vi "manual_trigger.vi"() -> ()   [LabVIEW 2011]
panel:
  in  "double trigger fast":bool
  in  "meas delay":u32
  in  "double trigger delayed":bool
  out "trigger number":i32
  in  "cont. trigger":bool
  in  "milliseconds to wait":u32=100
  in  "number of triggers":i32
  in  "single trigger":bool
  in  "stop":bool
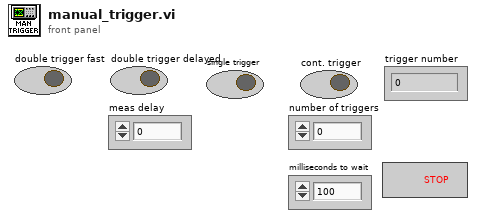
[diagram p1: front panel]
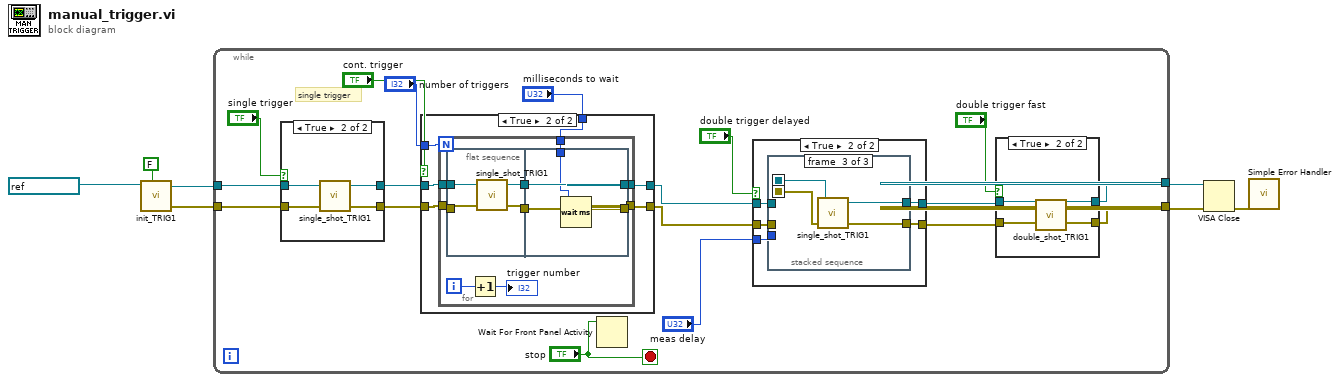
[diagram p0: block diagram]
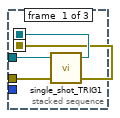
[diagram p4: hidden frame]
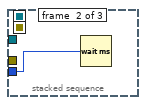
[diagram p5: hidden frame]
diagram:
  n1 = call "init_TRIG1.vi"("reset"=FALSE ("reset TRIG"), "VISA resource name"=refnum<visa-resource-name> "TRIG1") -> ("error out"=w6:errorcluster, "VISA resource name out"=w7:refnum<visa-resource-name>)  [unwired: 8 in]
  n2 = while {
    tunnel: w7 -> [w23]
    tunnel: w6 -> [w22]
    tunnel: [w10] -> w4
    tunnel: [w9] -> w3
    stop <- "stop" stop-if-true
    # "single trigger"
    n3 = case shown="True" "single trigger" {
      tunnel: w23 -> [w49 w53]
      tunnel: w22 -> [w48 w52]
      tunnel: [w49 w51] -> w21
      tunnel: [w48 w50] -> w20
      frame False {
      }
      frame True {
        n4 = call "single_shot_TRIG1.vi"("error in (no error)"=w52, "VISA resource name"=w53) -> ("error out"=w50:errorcluster, "VISA resource name 2"=w51:refnum<visa-resource-name>)  [unwired: 2 in]
      }
    }
    n5 = case shown="True" "cont. trigger" {
      tunnel: w21 -> [w55 w61]
      tunnel: w20 -> [w54 w60]
      tunnel: [w55 w59] -> w15
      tunnel: [w54 w58] -> w14
      tunnel: "number of triggers" -> [_ w57]
      tunnel: "milliseconds to wait" -> [_ w56]
      frame False {
      }
      frame True {
        n6 = for {
          N: w57 -> [_]
          tunnel: w61 -> [w70]
          tunnel: w60 -> [w69]
          tunnel: [w68] -> w59
          tunnel: [w67] -> w58
          tunnel: w56 -> [w64]
          i -> [w63]
          n7 = flat-sequence {
            tunnel: w70 -> [w74]
            tunnel: w69 -> [w73]
            tunnel: [w72] -> w66
            tunnel: [w71] -> w65
            tunnel: [w76] -> w67
            tunnel: [w77] -> w68
            tunnel: w66 -> [w77]
            tunnel: w65 -> [w76]
            tunnel: w64 -> [w75]
            frame #0 {
              n8 = call "single_shot_TRIG1.vi"("error in (no error)"=w73, "VISA resource name"=w74) -> ("error out"=w71:errorcluster, "VISA resource name 2"=w72:refnum<visa-resource-name>)  [unwired: 2 in]
            }
            frame #1 {
              n9 = Wait (ms)(milliseconds to wait=w75) -> ()  [unwired: 1 out]
            }
          }
          n10 = Increment(x=w63) -> (x+1=→"trigger number":i32)
        }
      }
    }
    n11 = Wait For Front Panel Activity(3:"stop") -> ()  [unwired: 2 in, 1 out]
    n12 = case shown="True" "double trigger delayed" {
      tunnel: w15 -> [w33 w38]
      tunnel: w14 -> [w32 w37]
      tunnel: [w33 w35] -> w12
      tunnel: [w32 w34] -> w11
      tunnel: "meas delay" -> [_ w36]
      frame False {
      }
      frame True {
        n13 = stacked-sequence {
          seq-local: [w40 _ _] -> [_ _ w46]
          seq-local: [w39 _ _] -> [_ _ w47]
          tunnel: w38 -> [w41 _ _]
          tunnel: w37 -> [w42 _ _]
          tunnel: w36 -> [_ w43 _]
          tunnel: [_ _ w45] -> w35
          tunnel: [_ _ w44] -> w34
          frame #0 {
            n14 = call "single_shot_TRIG1.vi"("error in (no error)"=w42, "VISA resource name"=w41) -> ("error out"=w39:errorcluster, "VISA resource name 2"=w40:refnum<visa-resource-name>)  [unwired: 2 in]
          }
          frame #1 {
            n15 = Wait (ms)(milliseconds to wait=w43) -> ()  [unwired: 1 out]
          }
          frame #2 {
            n16 = call "single_shot_TRIG1.vi"("error in (no error)"=w47, "VISA resource name"=w46) -> ("error out"=w44:errorcluster, "VISA resource name 2"=w45:refnum<visa-resource-name>)  [unwired: 2 in]
          }
        }
      }
    }
    n17 = case shown="True" "double trigger fast" {
      tunnel: w12 -> [w27 w31]
      tunnel: w11 -> [w26 w30]
      tunnel: [w27 w29] -> w10
      tunnel: [w26 w28] -> w9
      frame False {
      }
      frame True {
        n18 = call "double_shot_TRIG1.vi"("error in (no error)"=w30, "VISA resource name"=w31) -> ("error out"=w28:errorcluster, "VISA resource name 2"=w29:refnum<visa-resource-name>)  [unwired: 2 in]
      }
    }
  }
  n19 = VISA Close(VISA resource name=w4, error in (no error)=w3) -> (error out=w5:errorcluster)
  n20 = call <vilib>:"Simple Error Handler.vi"("error in (no error)"=w5) -> ()  [unwired: 4 in, 5 out]
